vi "Update Obj Calibration parameters to matlab script.vi"(8 "error in":errorcluster, 11 "Current Calibration Parameters":T1) -> (0 "error out":errorcluster)   [LabVIEW 2020]
uses:
  TypeDefs/Current Calibration Parameters.ctl
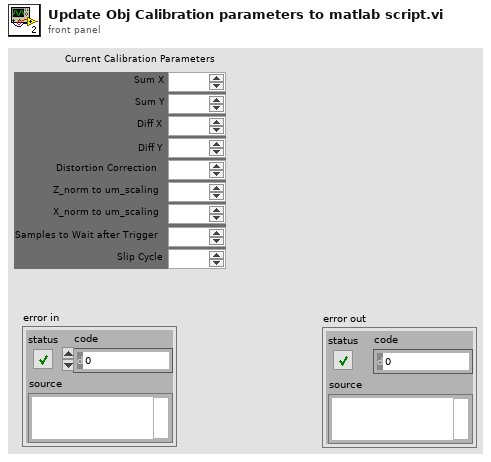
[diagram p1: front panel]
types:
  T1 = typedef "Current Calibration Parameters.ctl" = cluster{"Sum X":dbl, "Sum Y":dbl, "Diff X":dbl, "Diff Y":dbl, "Distortion Correction":dbl, "Z_norm to um_scaling":dbl, "X_norm to um_scaling":dbl, "Samples to Wait after Trigger":dbl, "Slip Cycle":dbl}
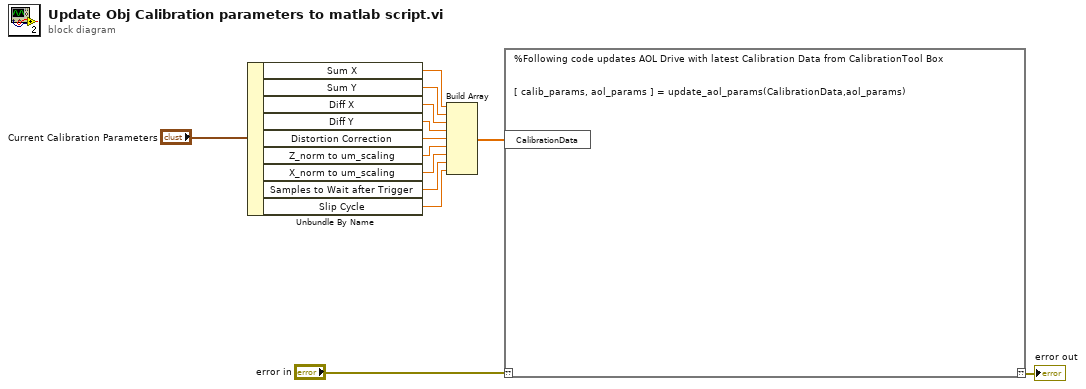
[diagram p0: block diagram]
diagram:
  n1 = Unbundle By Name("Current Calibration Parameters") -> ("Sum X"=w13:dbl, "Sum Y"=w12:dbl, "Diff X"=w11:dbl, "Diff Y"=w10:dbl, "Distortion Correction"=w9:dbl, "Z_norm to um_scaling"=w8:dbl, "X_norm to um_scaling"=w7:dbl, "Samples to Wait after Trigger"=w6:dbl, "Slip Cycle"=w5:dbl)
  n2 = Build Array(w13, w12, w11, w10, w9, w8, w7, w6, w5) -> (w4:dbl[])
  n3 = script code="%Following code updates AOL Drive with latest Calibration Data from CalibrationTool Box\n\n\n[ calib_params, aol_params ] = update_aol_params(CalibrationData,aol_params)"("??"="error in", "CalibrationData"=w4) -> ("??"=→"error out":errorcluster)
